vi "qIPR.vi"(0 "System no.":i32=1 min=1 max=4 step=1, 5 "error in":errorcluster) -> (14 "List of Interpreter Configurations":T1[](array[typedef]), 19 "error out":errorcluster)   [LabVIEW 2020]
doc: "IPR? (Get Interpreter)\n\nQueries the assignment of the currently used communication interface to a GCS interpreter.\n\nFormat\nIPR?\n\nArguments\nnone\n\nResponse\nEach communication interface of the controller is assigned to exactly one function unit \n\"Interpreter\" of type GCS. The response to IPR? has the following format:\nSYS_x INTPR_x\nSYS_x\nContainer unit from the \"System\" family\nx is the InstanceID of the container unit in the controller.\nAlias of the container unit \nINTPR_x\nFunction unit of type GCS from the \"Interpreter\" family\nx is the InstanceID of the function unit in the controller.\nAlias of the function unit \n\nExample\nFor the currently used communication interface, the supported user command levels are to be \nfound out. The user command levels are a property of the function units \"Interpreter\" of type \nGCS. Therefore, IPR? is first used to determine the GCS interpreter that is assigned to the \ncurrently used communication interface. Then USG? PROP is used to query the \nproperties of this GCS interpreter.\n>>IPR?\n<<SYS_1 INTPR_1\n>>USG? PROP SYS_1 INTPR_1\n<<#Unit Properties: <Container Unit> <Function Unit> \n<Description>\n<<SYS_1 INTPR_1 Interpreter of Type GCS\n<< #User Command Level: <Name> <Description>\n<< USR User Level\n<< ADV Expert Customer\n<< FAY Only PI Staff\n<< DEV Only FW Developer\n<< #END User Command Level\n<<#END Unit Properties\n\nUser command level\nUSR"
uses:
  InterpreterConfiguration.ctl
panel:
  # "IPR? (Get Interpreter)\n\nQueries the assignment of the currently used communication interface to a GCS interpreter."
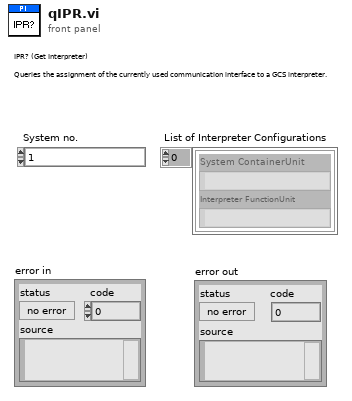
[diagram p1: front panel]
types:
  T1 = typedef "InterpreterConfiguration.ctl" = cluster{"System ContainerUnit":string, "Interpreter FunctionUnit":string}
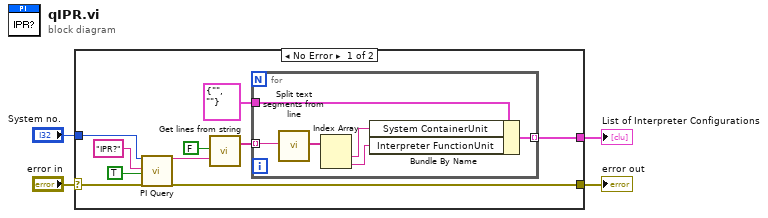
[diagram p0: block diagram]
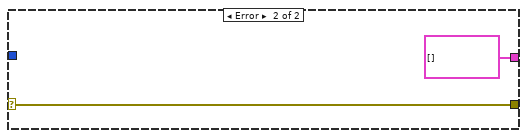
[diagram p2: hidden frame]
diagram:
  n1 = case shown="No Error" "error in" {
    selector: "error in" -> [w11 w22]
    tunnel: [w10 w22] -> w4
    tunnel: "System no." -> [w14 _]
    tunnel: [w5 T1[] [] ("List of Interpreter Configurations")] -> w1
    frame No Error {
      n2 = call "PI Query.vi"("System no."=w14, "String to send"="IPR?", "Attach termination char.?"=TRUE, "error in"=w11) -> ("String read"=w9:string, "error out"=w10:errorcluster)  [unwired: 3 in, 11 out]
      n3 = call "Get lines from string.vi"("Cut spaces?"=FALSE, "Input string"=w9) -> ("Strings"=w8:string[])  [unwired: 16 in, 1 out]
      n4 = for {
        tunnel: w8 -> [w20] mode=indexing
        tunnel: T1 {"System ContainerUnit"="", "Interpreter FunctionUnit"=""} ("InterpreterConfiguration") -> [w19]
        tunnel: [w15] -> w5 mode=indexing
        n5 = call "Split text segments from line.vi"("Input line string"=w20) -> ("Text segments"=w18:string[])  [unwired: 18 in]
        n6 = Index Array(array=w18) -> (element #1=w17:string, element #2=w16:string)  [unwired: 2 in]
        n7 = Bundle By Name(cluster=w19, "System ContainerUnit"=w17, "Interpreter FunctionUnit"=w16) -> (w15:T1)
      }
    }
    frame Error {
    }
  }
  "error out" <- w4
  "List of Interpreter Configurations" <- w1
